vi "EyeBlinkConditioning.vi"() -> ()   [LabVIEW 2013]
uses:
  <vilib>/Platform/TimedLoop/XDataNode/timing_clust.ctl
  <vilib>/Platform/TimedLoop/XDataNode/nitl_modes.ctl
  <vilib>/Platform/TimedLoop/XDataNode/wakeup.ctl
  <vilib>/Analysis/1siggen.llb/Riffle Array (DBL).vi
  <vilib>/Utility/file.llb/Write To Spreadsheet File (string).vi
  <vilib>/platform/TimedLoop/XDataNode/XDataNode.xnode
  <vilib>/Platform/TimedLoop/XDataNode/XDNodeRunTimeDep.lvlib
  <vilib>/Analysis/NI_AALBase.lvlib
panel:
  out "Stimulus order":dbl[](array[numeric])
  out "next trial":string
  out "CS Trial indexs & time":string[][](array[string])
  out "US (Air Puff)":bool
  out "CS (Tone)":bool
  out "Total trial/session":i32
  in  "Mouse ID":string="Q4#09"
  in  "file path (dialog if empty)":path=path "C:/Users/George Augustine Lab/Helen-treadmill/pmr-Helen/EyeBlinkConditioning/EyeBlink_Data/20220515/20220515_EyeBlink1KTone_Q4#09"
  out "current trial duration (ms)":dbl
  in  "stop task":bool
  out "Task Duration (min)":dbl
  out "No. of Trials":dbl
  out "ITI (s) [next-current]":dbl
  # "1 -- paired\n0 -- CS only\n#First 30 trials are always paired\n#The last 60 trials have 10 CR only randomly inserted\n#CS randomly & non-continuously appear \n\n#ITI is randomly between 25s and 35s\n#Delay between CS and US is 250ms\n#CS--500ms (total); US--50ms (total)"
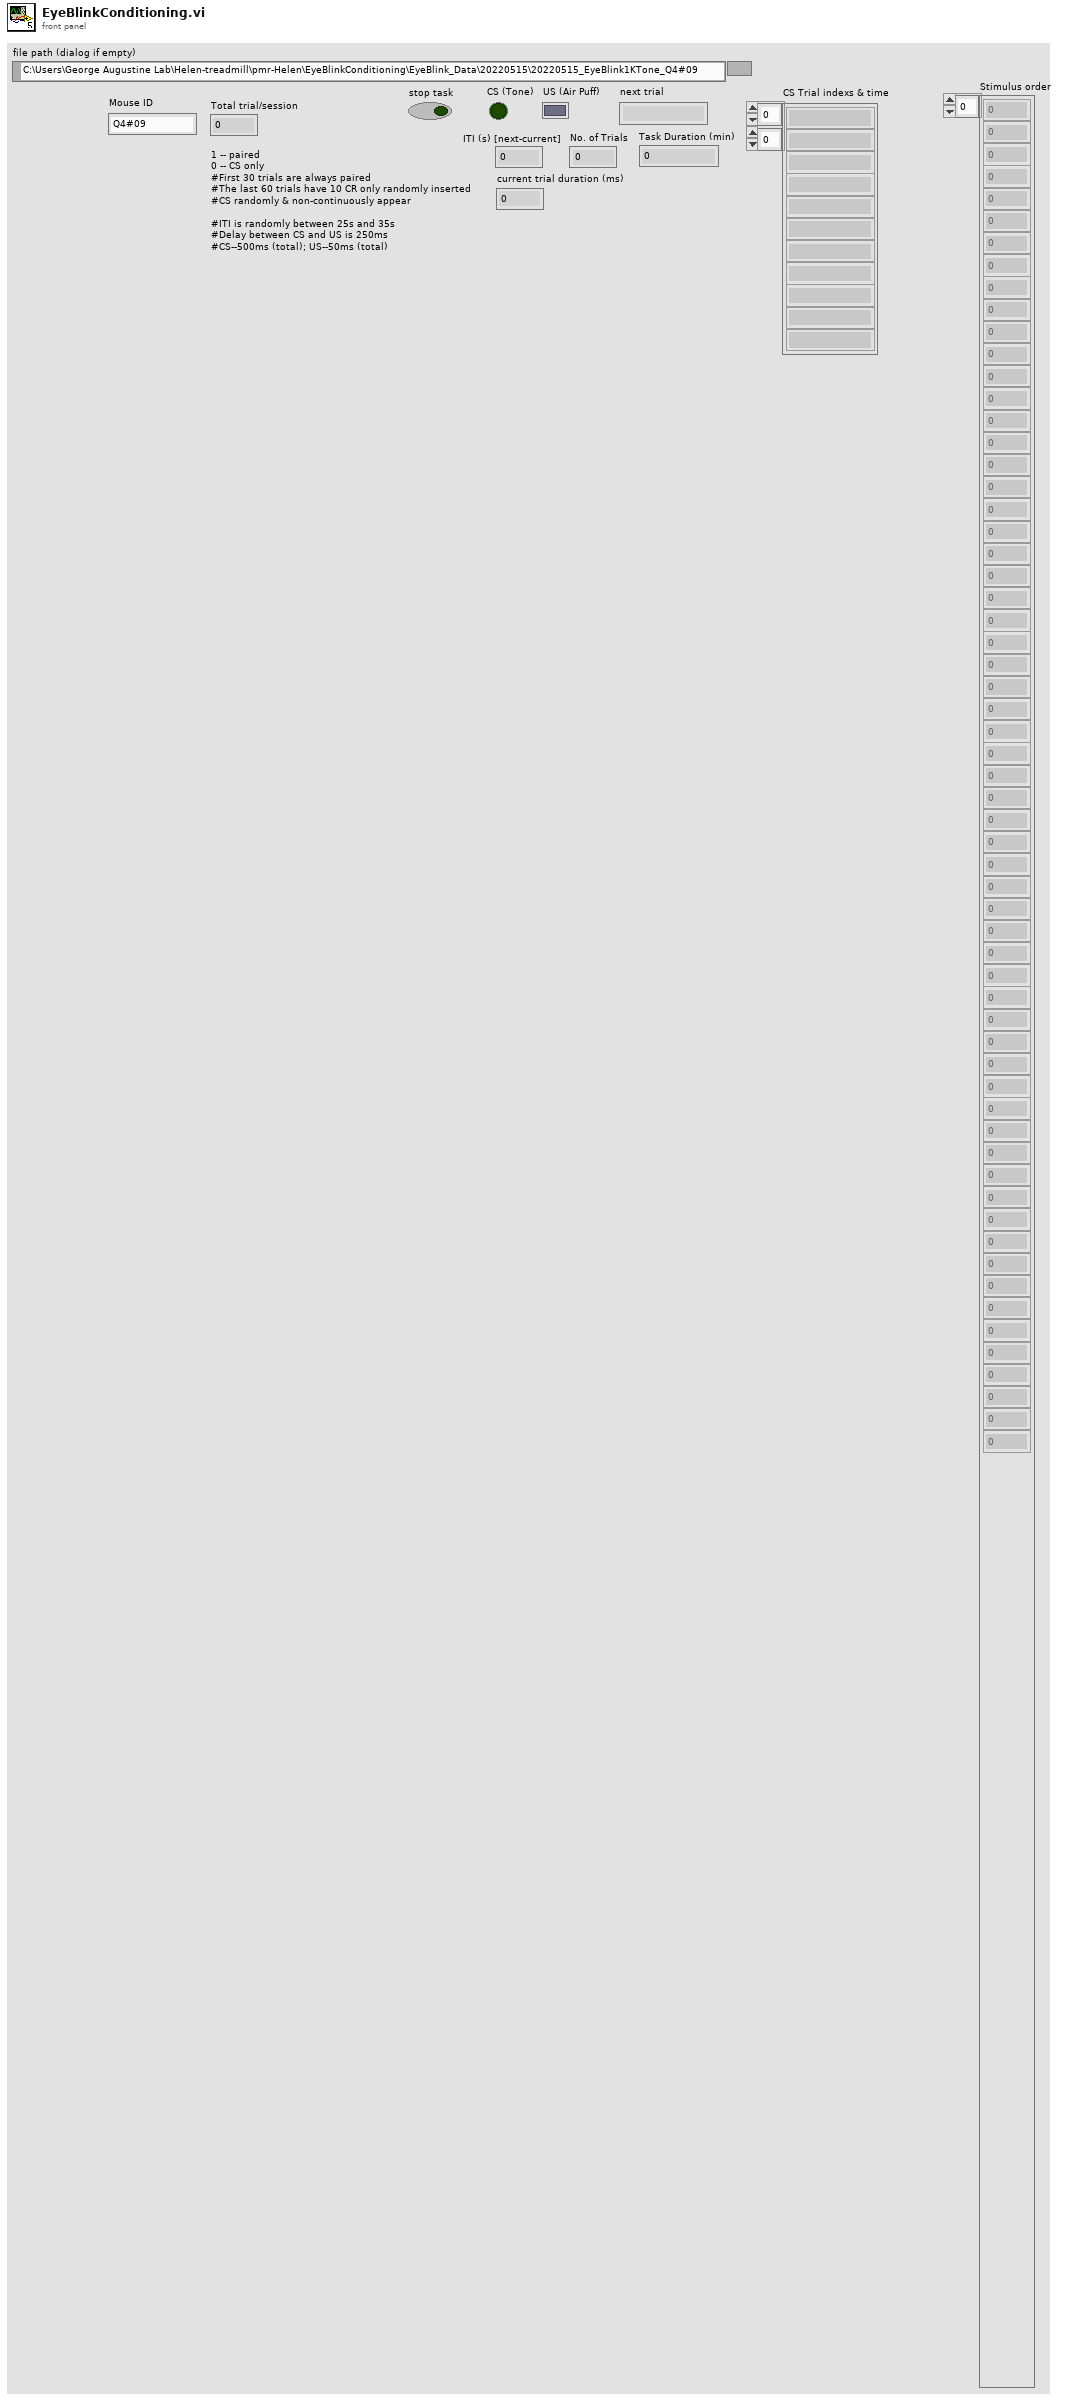
[diagram p1: front panel]
types:
  T1 = typedef "XDNodeRunTimeDep.lvlib/timing_clust.ctl" = cluster{"Expected End [f-1]":u64, "Actual End [f-1]":u64, "Finished Late? [f-1]":bool, "Expected End [i-1]":u64, "Actual End [i-1]":u64, "Finished Late? [i-1]":bool, "Expected Start [i]":u64, "Actual Start [i]":u64, "Expected Start [f]":u64, "Actual Start [f]":u64, "Source Name":string, "Structure Name":string, "Period":i64, "Deadline":i64, "Offset":i64, "Start":i64, "Priority":i32, "Timeout":i32, "Mode":T2, "Wakeup Reason":T3, "Error":errorcluster, "Source Type":string, "Secondary Source Type":string, "Global End Time":u64, "Global Start Time":u64, "Frame Duration":u64, "Iteration Duration":u64, "Assigned CPU":i32, "I/O Scan Engine Mode":u32}
  T2 = typedef "XDNodeRunTimeDep.lvlib/nitl_modes.ctl" = enum32{"No Change", "Process missed periods, maintain original phase", "Discard missed periods, maintain original phase", "Process missed periods, ignore original phase", "Discard missed periods, ignore original phase"}
  T3 = typedef "XDNodeRunTimeDep.lvlib/wakeup.ctl" = enum32{"Normal", "Aborted", "Asynchronous wakeup", "Timing source error", "Timed loop error", "Timeout"}
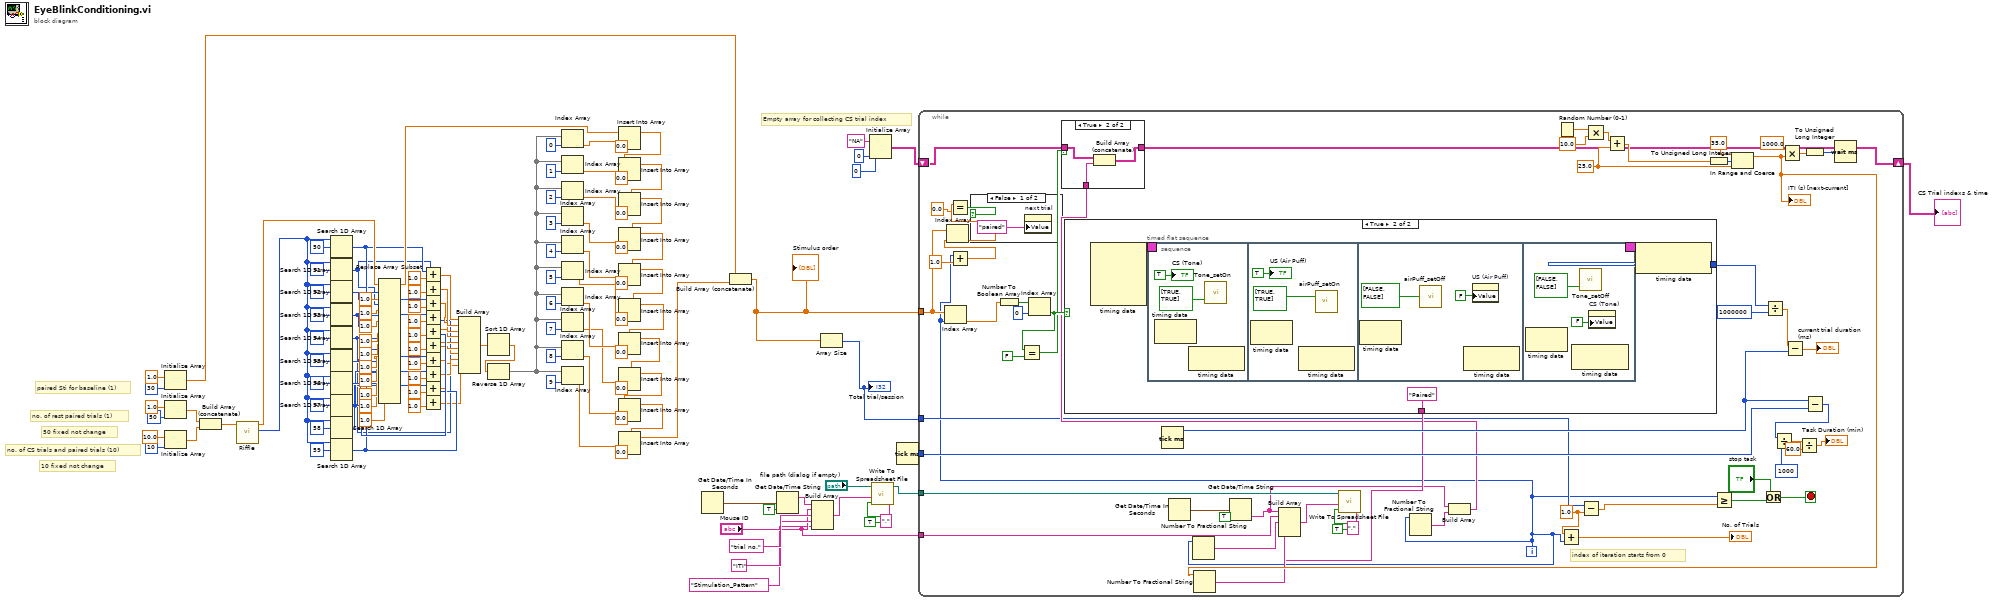
[diagram p0: block diagram]
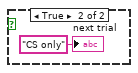
[diagram p2: hidden frame]
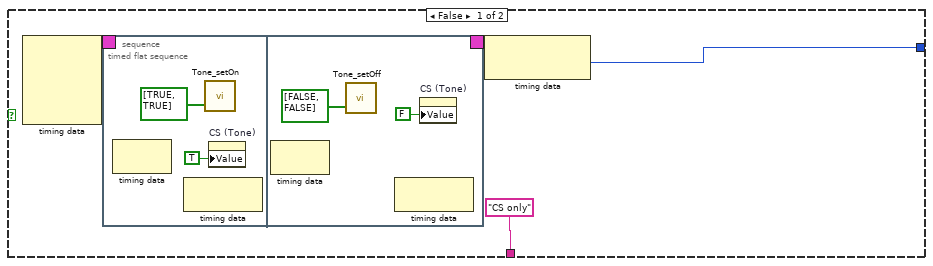
[diagram p4: hidden frame]
diagram:
  # "50 fixed not change"
  # "10 fixed not change"
  # "no. of rest paired trials (1)"
  # "no. of CS trials and paired trials (10)"
  # "paired Sti for baseline (1)"
  # "Empty array for collecting CS trial index"
  n1 = Initialize Array(1.0 ("element"), 30 ("dimension size")) -> (w94:dbl[])
  n2 = Initialize Array(1.0 ("element"), 50 ("dimension size")) -> (w98:dbl[])
  n3 = Initialize Array(10.0 ("element"), 10 ("dimension size")) -> (w99:dbl[])
  n4 = Build Array (concatenate)(w98, w99) -> (w97:dbl[])
  n5 = call-poly <vilib>:"Riffle.vi"("X"=w97) -> ("Riffled Index"=w107:i32[], "Riffled {X}"=w106:dbl[])  [unwired: 8 in, 1 out]
  n6 = Search 1D Array(1D array=w107, element=50) -> (index of element=w44:i32)  [unwired: 1 in]
  n7 = Search 1D Array(1D array=w107, element=51) -> (index of element=w43:i32)  [unwired: 1 in]
  n8 = Search 1D Array(1D array=w107, element=52) -> (index of element=w42:i32)  [unwired: 1 in]
  n9 = Search 1D Array(1D array=w107, element=53) -> (index of element=w41:i32)  [unwired: 1 in]
  n10 = Search 1D Array(1D array=w107, element=54) -> (index of element=w27:i32)  [unwired: 1 in]
  n11 = Search 1D Array(1D array=w107, element=55) -> (index of element=w40:i32)  [unwired: 1 in]
  n12 = Search 1D Array(1D array=w107, element=56) -> (index of element=w39:i32)  [unwired: 1 in]
  n13 = Search 1D Array(1D array=w107, element=57) -> (index of element=w38:i32)  [unwired: 1 in]
  n14 = Search 1D Array(1D array=w107, element=58) -> (index of element=w37:i32)  [unwired: 1 in]
  n15 = Search 1D Array(1D array=w107, element=59) -> (index of element=w36:i32)  [unwired: 1 in]
  n16 = Replace Array Subset(array=w106, new element #1=1.0 ("new element/subarray"), index #1=w44, new element #2=1.0 ("new element/subarray"), index #2=w43, new element #3=1.0 ("new element/subarray"), index #3=w42, new element #4=1.0 ("new element/subarray"), index #4=w41, new element #5=1.0 ("new element/subarray"), index #5=w27, new element #6=1.0 ("new element/subarray"), index #6=w40, new element #7=1.0 ("new element/subarray"), index #7=w39, new element #8=1.0 ("new element/subarray"), index #8=w38, new element #9=1.0 ("new element/subarray"), index #9=w37, new element #10=1.0 ("new element/subarray"), index #10=w36) -> (w104:dbl[])
  n17 = Add(x=w44, y=1.0) -> (x+y=w53:dbl)
  n18 = Add(x=w43, y=1.0) -> (x+y=w35:dbl)
  n19 = Add(x=w42, y=1.0) -> (x+y=w34:dbl)
  n20 = Add(x=w41, y=1.0) -> (x+y=w33:dbl)
  n21 = Add(x=w27, y=1.0) -> (x+y=w32:dbl)
  n22 = Add(x=w40, y=1.0) -> (x+y=w31:dbl)
  n23 = Add(x=w39, y=1.0) -> (x+y=w30:dbl)
  n24 = Add(x=w38, y=1.0) -> (x+y=w29:dbl)
  n25 = Add(x=w37, y=1.0) -> (x+y=w28:dbl)
  n26 = Add(x=w36, y=1.0) -> (x+y=w26:dbl)
  n27 = Build Array(w53, w35, w34, w33, w32, w31, w30, w29, w28, w26) -> (w14:dbl[])
  n28 = Sort 1D Array(array=w14) -> (sorted array=w25:dbl[])
  n29 = Reverse 1D Array(array=w25) -> (reversed array=w12:dbl[])
  n30 = Index Array(array=w12, index=0) -> (element=w13:dbl)
  n31 = Index Array(array=w12, index=1) -> (element=w11:dbl)
  n32 = Index Array(array=w12, index=2) -> (element=w10:dbl)
  n33 = Index Array(array=w12, index=3) -> (element=w9:dbl)
  n34 = Index Array(array=w12, index=4) -> (element=w7:dbl)
  n35 = Index Array(array=w12, index=5) -> (element=w6:dbl)
  n36 = Index Array(array=w12, index=6) -> (element=w5:dbl)
  n37 = Index Array(array=w12, index=7) -> (element=w4:dbl)
  n38 = Index Array(array=w12, index=8) -> (element=w3:dbl)
  n39 = Index Array(array=w12, index=9) -> (element=w2:dbl)
  n40 = Insert Into Array(array=w104, index=w13, new element=0.0 ("new element/subarray")) -> (w71:dbl[])
  n41 = Insert Into Array(array=w71, index=w11, new element=0.0 ("new element/subarray")) -> (w69:dbl[])
  n42 = Insert Into Array(array=w69, index=w10, new element=0.0 ("new element/subarray")) -> (w67:dbl[])
  n43 = Insert Into Array(array=w67, index=w9, new element=0.0 ("new element/subarray")) -> (w66:dbl[])
  n44 = Insert Into Array(array=w66, index=w7, new element=0.0 ("new element/subarray")) -> (w65:dbl[])
  n45 = Insert Into Array(array=w65, index=w6, new element=0.0 ("new element/subarray")) -> (w58:dbl[])
  n46 = Insert Into Array(array=w58, index=w5, new element=0.0 ("new element/subarray")) -> (w57:dbl[])
  n47 = Insert Into Array(array=w57, index=w4, new element=0.0 ("new element/subarray")) -> (w61:dbl[])
  n48 = Insert Into Array(array=w61, index=w3, new element=0.0 ("new element/subarray")) -> (w56:dbl[])
  n49 = Insert Into Array(array=w56, index=w2, new element=0.0 ("new element/subarray")) -> (w105:dbl[])
  n50 = Get Date/Time In Seconds() -> (seconds since 1Jan1904=w121:timestamp)
  n51 = Build Array (concatenate)(w94, w105) -> (w1:dbl[])
  "Stimulus order" <- w1
  n52 = Get Date/Time String(seconds (now)=w121, want seconds? (F)=TRUE) -> (date string=w120:string)  [unwired: 1 in, 1 out]
  n53 = Build Array(w120, "Mouse ID", "trial no." ("element"), "ITI" ("element"), "Stimulation_Pattern" ("element")) -> (w117:string[])
  n54 = Array Size(array=w1) -> (size(s)=w114:i32)
  "Total trial/session" <- w114
  n55 = Initialize Array("NA" ("element"), 0 ("dimension size"), 0 ("dimension size")) -> (w109:string[][])
  n56 = call-poly <vilib>:"Write To Spreadsheet File.vi"("delimiter (\\t)"="," ("delimiter (\\t)"), "append to file? (new file:F)"=TRUE, "1D data"=w117, "file path (dialog if empty)"="file path (dialog if empty)") -> ("new file path (Not A Path if cancelled)"=w116:path)  [unwired: 4 in]
  n57 = Tick Count (ms)() -> (millisecond timer value=w126:u32)
  n58 = while {
    tunnel: w126 -> [w167]
    tunnel: w116 -> [w158]
    tunnel: "Mouse ID" -> [w157]
    tunnel: w1 -> [w137]
    tunnel: w114 -> [w131]
    shift-right: [w141] -> w108
    shift-left: w109 -> [w146]
    i -> [w127]
    stop <- w173 stop-if-true
    w129 = 1.0 ("y")
    w181 = 25.0 ("Randomized ITI between (s)")
    # "index of iteration starts from 0"
    n59 = Index Array(array=w137, index=w127) -> (element=w150:dbl)
    n60 = Add(x=w127, y=1.0) -> (x+y=w135:dbl)
    n61 = Index Array(array=w137, index=w135) -> (element=w133:dbl)
    n62 = Equal?(x=w133, y=0.0) -> (x = y?=w134:bool)
    n63 = case shown="False" w134 {
      frame False {
        n64 = property on="next trial" class="Str"("Value"="paired" ("next trial")) -> ()  [unwired: 2 in, 2 out]
      }
      frame True {
        "next trial" <- "CS only" ("next trial")
      }
    }
    n65 = Number To Boolean Array(number=w150) -> (Boolean array=w152:bool[])
    n66 = Index Array(array=w152, index=0) -> (element=w148:bool)
    n67 = Equal?(x=w148, y=FALSE) -> (x = y?=w145:bool)
    n68 = case shown="True" w148 {
      tunnel: [w191 w206] -> w153
      tunnel: ["CS only" "Paired"] -> w149
      frame False {
        n69 = node-c288() -> (w193:T1)  [unwired: 4 in]
        n70 = timed-sequence {
          timing: w193 -> [_]
          timing-out: [_] -> w192
          n71 = timed-flat-sequence {
            frame #0 {
              n72 = node-c288() -> ()  [unwired: 1 in, 1 out]
              n73 = node-c288() -> ()  [unwired: 1 in, 1 out]
              n74 = call "Tone_setOn"("data"=bool[] [TRUE, TRUE]) -> ()  [unwired: 17 in, 2 out]
              n75 = property on="CS (Tone)" class="Bool (strict)"("Value"=TRUE ("CS (LED)")) -> ()  [unwired: 2 in, 2 out]
            }
            frame #1 {
              n76 = node-c288() -> ()  [unwired: 1 in, 1 out]
              n77 = call "Tone_setOff"("data"=bool[] [FALSE, FALSE]) -> ()  [unwired: 17 in, 2 out]
              n78 = node-c288() -> ()  [unwired: 1 in, 1 out]
              n79 = property on="CS (Tone)" class="Bool (strict)"("Value"=FALSE ("CS (LED)")) -> ()  [unwired: 2 in, 2 out]
            }
          }
        }
        n80 = node-c288(w192) -> (w191:i64)
      }
      frame True {
        n81 = node-c288() -> (w208:T1)  [unwired: 4 in]
        n82 = timed-sequence {
          timing: w208 -> [_]
          timing-out: [_] -> w207
          n83 = timed-flat-sequence {
            frame #0 {
              n84 = node-c288() -> ()  [unwired: 1 in, 1 out]
              n85 = node-c288() -> ()  [unwired: 1 in, 1 out]
              n86 = call "Tone_setOn"("data"=bool[] [TRUE, TRUE]) -> ()  [unwired: 17 in, 2 out]
              "CS (Tone)" <- TRUE ("CS (LED)")
            }
            frame #1 {
              n87 = node-c288() -> ()  [unwired: 1 in, 1 out]
              n88 = node-c288() -> ()  [unwired: 1 in, 1 out]
              n89 = call "airPuff_setOn"("data"=bool[] [TRUE, TRUE]) -> ()  [unwired: 17 in, 2 out]
              "US (Air Puff)" <- TRUE ("US (Air Puff)")
            }
            frame #2 {
              n90 = node-c288() -> ()  [unwired: 1 in, 1 out]
              n91 = call "airPuff_setOff"("data"=bool[] [FALSE, FALSE]) -> ()  [unwired: 17 in, 2 out]
              n92 = node-c288() -> ()  [unwired: 1 in, 1 out]
              n93 = property on="US (Air Puff)" class="Bool (strict)"("Value"=FALSE ("US (Air Puff)")) -> ()  [unwired: 2 in, 2 out]
            }
            frame #3 {
              n94 = node-c288() -> ()  [unwired: 1 in, 1 out]
              n95 = node-c288() -> ()  [unwired: 1 in, 1 out]
              n96 = call "Tone_setOff"("data"=bool[] [FALSE, FALSE]) -> ()  [unwired: 17 in, 2 out]
              n97 = property on="CS (Tone)" class="Bool (strict)"("Value"=FALSE ("CS (LED)")) -> ()  [unwired: 2 in, 2 out]
            }
          }
        }
        n98 = node-c288(w207) -> (w206:i64)
      }
    }
    n99 = Tick Count (ms)() -> (millisecond timer value=w166:u32)
    n100 = Get Date/Time In Seconds() -> (seconds since 1Jan1904=w162:timestamp)
    n101 = Number To Fractional String(number=w127) -> (F-format string=w154:string)  [unwired: 3 in]
    n102 = Get Date/Time String(seconds (now)=w162, want seconds? (F)=TRUE) -> (time string=w143:string)  [unwired: 1 in, 1 out]
    n103 = Number To Fractional String(number=w127) -> (F-format string=w144:string)  [unwired: 3 in]
    n104 = Build Array(w143, w144) -> (w142:string[])
    n105 = case shown="True" w145 {
      tunnel: w146 -> [w186 w189]
      tunnel: w142 -> [_ w188]
      tunnel: [w186 w187] -> w141
      frame False {
      }
      frame True {
        n106 = Build Array (concatenate)(w189, w188) -> (w187:string[][])
      }
    }
    n107 = Random Number (0-1)() -> (number: 0 to 1=w179:dbl)
    n108 = Add(x=w129, y=w127) -> (x+y=→"No. of Trials":dbl)
    n109 = Subtract(x=w131, y=w129) -> (x-y=w130:dbl)
    n110 = Multiply(x=w179, y=10.0) -> (x*y=w180:dbl)
    n111 = Add(x=w180, y=w181) -> (x+y=w182:dbl)
    n112 = To Unsigned Long Integer(number=w182) -> (unsigned 32bit integer=w178:u32)
    n113 = Greater Or Equal?(x=w127, y=w130) -> (x >= y?=w172:bool)
    n114 = In Range and Coerce(upper limit=35.0 ("And (s)"), x=w178, lower limit=w181) -> (coerced(x)=w156:dbl)  [unwired: 1 out]
    "ITI (s) [next-current]" <- w156
    n115 = Number To Fractional String(number=w156) -> (F-format string=w155:string)  [unwired: 3 in]
    n116 = Build Array(w143, w157, w154, w155, w149) -> (w163:string[])
    n117 = call-poly <vilib>:"Write To Spreadsheet File.vi"("delimiter (\\t)"="," ("delimiter (\\t)"), "append to file? (new file:F)"=TRUE, "1D data"=w163, "file path (dialog if empty)"=w158) -> ()  [unwired: 4 in, 1 out]
    n118 = Or(x="stop task", y=w172) -> (x .or. y?=w173:bool)
    n119 = Divide(x=w153, y=i64 1000000) -> (x/y=w164:dbl)
    n120 = Multiply(x=1000.0, y=w156) -> (x*y=w175:dbl)
    n121 = Subtract(x=w164, y=w166) -> (x-y=→"current trial duration (ms)":dbl)
    n122 = To Unsigned Long Integer(number=w175) -> (unsigned 32bit integer=w174:u32)
    n123 = Subtract(x=w166, y=w167) -> (x-y=w169:u32)
    n124 = Divide(x=w169, y=u32 1000) -> (x/y=w140:dbl)
    n125 = Divide(x=w140, y=60.0) -> (x/y=→"Task Duration (min)":dbl)
    n126 = Wait (ms)(milliseconds to wait=w174) -> ()  [unwired: 1 out]
  }
  "CS Trial indexs & time" <- w108
